vi "save calibration.vi"(7 "conversion in":T1={"conversion matrix"=[[0.0, 0.0], [0.0, 0.0], [0.0, 0.0], [0.0, 0.0], [0.0, 0.0], [0.0, 0.0]], "units"="", "name"="", "scale type"=enum."Volts", "offset (volts)"=0.0, "second channel"=0, "correspondence table"=[], "offset (physical units)"=0.0, "pH scale"={"Buffers"=[], "Temperature"=0.0}, "D.O."={"Temperature"=0.0, "K"=0.0, "barometric pressure"=0.0}} {"D.O."."K" format="%.6f"; "D.O."."Temperature" format="%.2f"; "pH scale"."Buffers"."V/T" format="%.5f"; "pH scale"."Buffers"."Buffer" format="%.2f"; "pH scale"."Temperature" format="%.2f"; "offset (physical units)" format="%.5f"; "correspondence table"."volts" format="%.4f"; "correspondence table"."physical units" format="%.4f"; "second channel" min=-1; "offset (volts)" format="%.5f"; "conversion matrix" format="%.4e"}) -> (3 "conversion out":T1={"conversion matrix"=[[0.0, 0.0], [0.0, 0.0], [0.0, 0.0], [0.0, 0.0], [0.0, 0.0], [0.0, 0.0]], "units"="", "name"="", "scale type"=enum."Volts", "offset (volts)"=0.0, "second channel"=0, "correspondence table"=[], "offset (physical units)"=0.0, "pH scale"={"Buffers"=[], "Temperature"=0.0}, "D.O."={"Temperature"=0.0, "K"=0.0, "barometric pressure"=0.0}} {"D.O."."K" format="%.6f"; "D.O."."Temperature" format="%.2f"; "pH scale"."Buffers"."V/T" format="%.5f"; "pH scale"."Buffers"."Buffer" format="%.2f"; "pH scale"."Temperature" format="%.2f"; "offset (physical units)" format="%.5f"; "correspondence table"."volts" format="%.4f"; "correspondence table"."physical units" format="%.4f"; "second channel" min=-1; "offset (volts)" format="%.5f"; "conversion matrix" format="%.4e"})   [LabVIEW 2010]
uses:
  calibration/conversion.ctl
  DAQ configuration/scale type.ctl
  calibration/correspondence table.ctl
  calibration/pH/pH scale.ctl
  calibration/Dissolved Oxygen/DO scale.ctl
panel:
  out "?":errorcluster
  # "C"
  # "kPa"
  # "C"
  # "C"
  # "kPa"
  # "C"
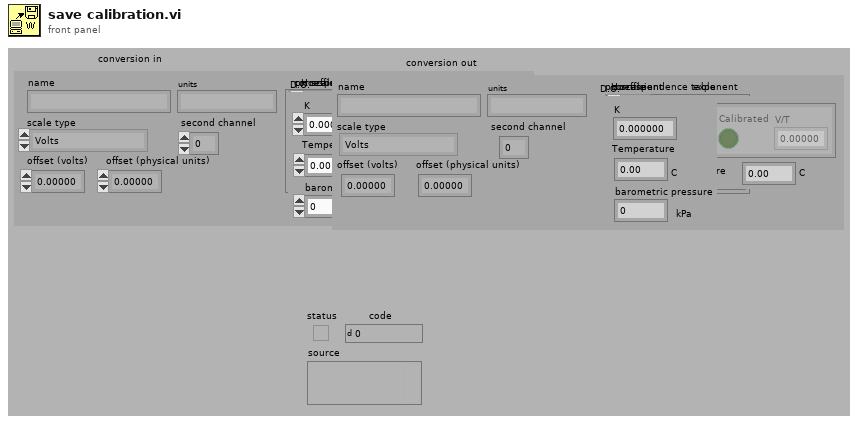
[diagram p1: front panel]
types:
  T1 = typedef "conversion.ctl" = cluster{"conversion matrix":sgl[][], "units":string, "name":string, "scale type":T2, "offset (volts)":dbl, "second channel":i8, "correspondence table":T3, "offset (physical units)":dbl, "pH scale":T4, "D.O.":T5}
  T2 = typedef "scale type.ctl" = enum16{"Volts", "Polynomial", "Correspondence Table", "pH", "Dissolved Oxygen", "Quadratic"}
  T3 = typedef "correspondence table.ctl" = cluster{"physical units":dbl, "volts":dbl}[]
  T4 = typedef "pH scale.ctl" = cluster{"Buffers":cluster{"Buffer":dbl, "Calibrated":bool, "V/T":dbl}[], "Temperature":dbl}
  T5 = typedef "DO scale.ctl" = cluster{"Temperature":dbl, "K":dbl, "barometric pressure":dbl}
  T6 = enum16{"open", "open or create", "create or replace", "create", "open (read only)"}
  T7 = enum16{"open", "replace", "create", "open or create", "replace or create", "replace or create with confirmation"}
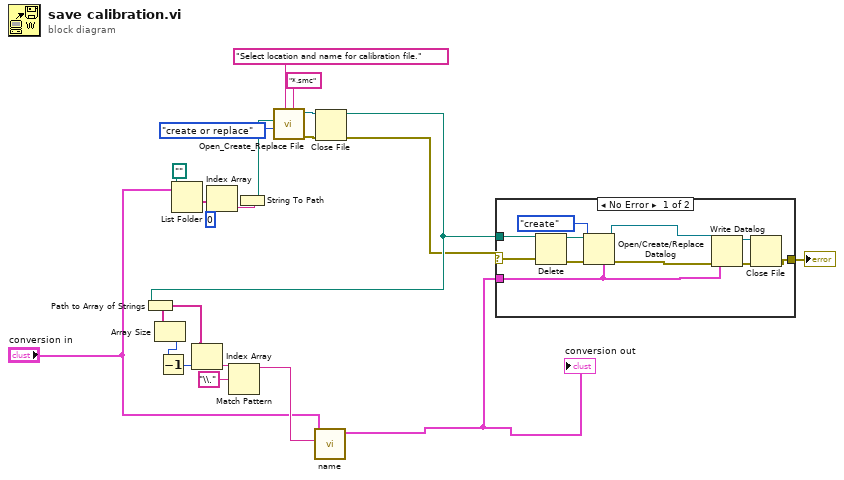
[diagram p0: block diagram]
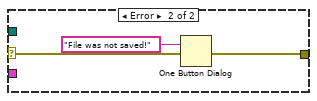
[diagram p2: hidden frame]
diagram:
  n1 = List Folder(datalog type="conversion in", path=path "") -> (folder names=w21:string[])  [unwired: 2 in, 3 out]
  n2 = Index Array(array=w21, index=0) -> (element=w19:string)
  n3 = String To Path(string=w19) -> (path=w4:path)
  n4 = call <vilib>:"Open_Create_Replace File.vi"("pattern"="*.smc", "prompt"="Select location and name for calibration file.", "function (open:0)"=T6."create or replace", "start path  (Not A Path)"=w4) -> ("error out"=w7:errorcluster, "refnum"=w6:refnum<file>)  [unwired: 4 in, 2 out]
  n5 = Close File(refnum=w6, error in=w7) -> (path=w2:path, error out=w1:errorcluster)
  n6 = Path to Array of Strings(0:w2) -> (2:w17:string[])  [unwired: 1 out]
  n7 = Array Size(array=w17) -> (size(s)=w16:i32)
  n8 = Decrement(x=w16) -> (x-1=w14:i32)
  n9 = Index Array(array=w17, index=w14) -> (element=w15:string)
  n10 = Match Pattern(string=w15, regular expression="\\.") -> (before substring=w12:string)  [unwired: 1 in, 3 out]
  n11 = call "name.vi"("name"=w12, "Scale in"="conversion in") -> ("Scale out"=w10:T1)  [unwired: 8 in]
  "conversion out" <- w10
  n12 = case shown="No Error" w1 {
    selector: w1 -> [w26 w33]
    tunnel: w2 -> [w24 _]
    tunnel: w10 -> [w29 _]
    tunnel: [w30 w33] -> w3
    frame No Error {
      n13 = Delete(path (use dialog)=w24, error in=w26) -> (deleted path=w23:path, error out=w25:errorcluster)  [unwired: 3 in, 1 out]
      n14 = Open/Create/Replace Datalog(5:w29, 8:w25, 10:T7."create" ("operation (0:open)"), 11:w23) -> (0:w27:errorcluster, 3:w28:refnum<k1>)  [unwired: 2 in, 1 out]
      n15 = Write Datalog(4:w27, 6:w29, 7:w28) -> (0:w32:errorcluster, 3:w31:refnum<k1>)
      n16 = Close File(refnum=w31, error in=w32) -> (error out=w30:errorcluster)  [unwired: 1 out]
    }
    frame Error {
      n17 = One Button Dialog(message="File was not saved!") -> ()  [unwired: 1 in, 1 out]
    }
  }
  "?" <- w3
